vi "Update State Data.vi"(8 "error in (no error)":errorcluster, 9 "Data":variant, 10 "Argument":string, 11 "String Assertion in":refnum<class "String Assertion.lvclass">) -> (0 "error out":errorcluster, 3 "String Assertion out":refnum<class "String Assertion.lvclass">)   [LabVIEW 2020, in "MacroAssert.lvlib" / "String Assertion.lvclass"]
uses:
  String Assertion.lvclass
  String Assertion Type.ctl
  String Comparator.ctl
  Assertion Step/Assertion Step.lvclass
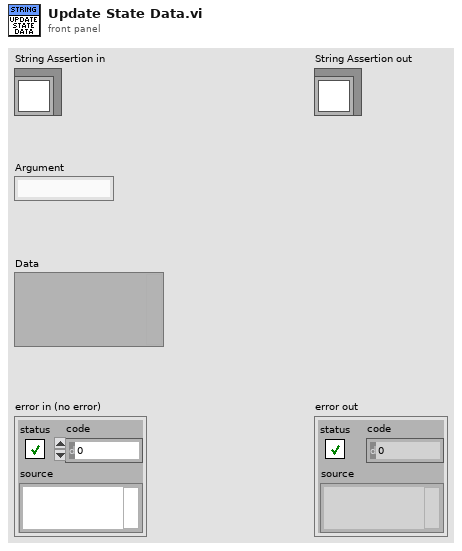
[diagram p1: front panel]
types:
  T1 = typedef "MacroAssert.lvlib/String Assertion.lvclass/String Assertion Type.ctl" = enum16{"String Ctl Value", "Ctl Caption Property", "Ctl Tip Strip Property", "Frontmost Window Name", "Frontmost VI Name"}
  T2 = typedef "MacroAssert.lvlib/String Assertion.lvclass/String Comparator.ctl" = enum16{"Contains", "Equals", "Starts with", "Ends with", "Does not contain", "Does not equal"}
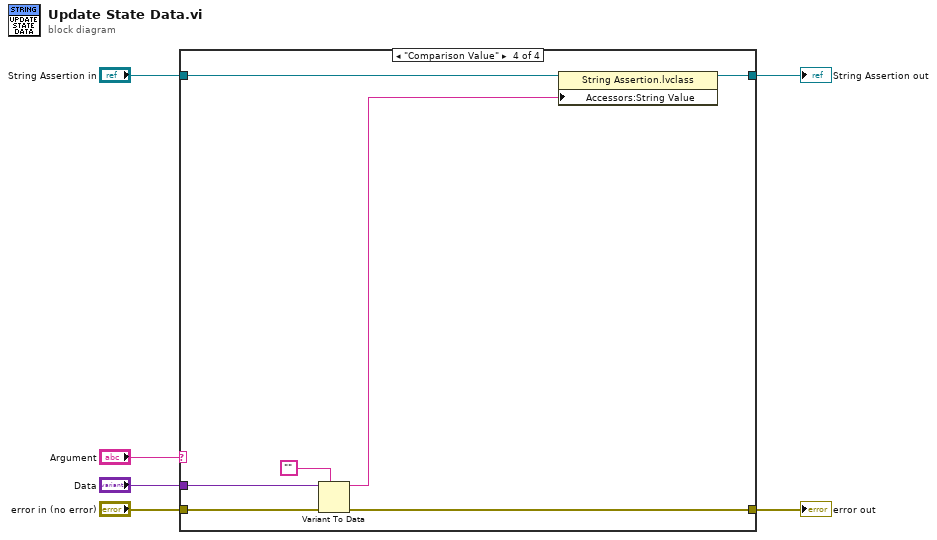
[diagram p0: block diagram]
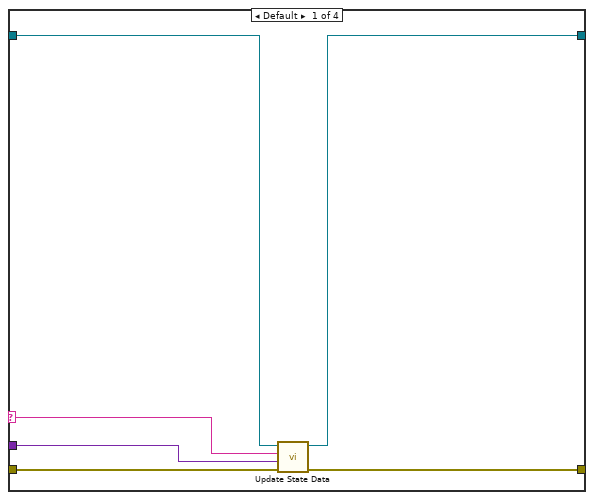
[diagram p2: hidden frame]
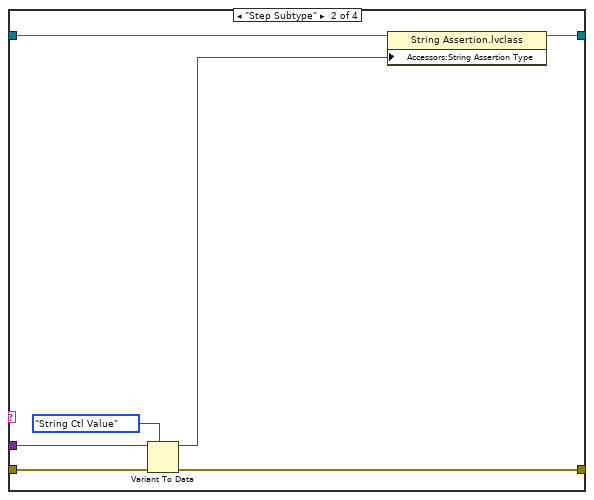
[diagram p3: hidden frame]
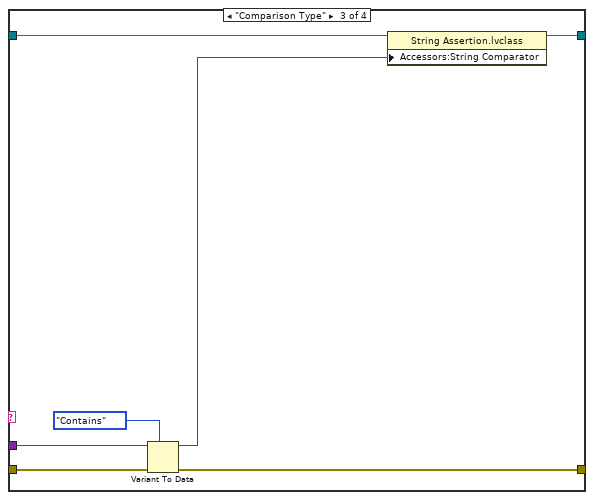
[diagram p4: hidden frame]
diagram:
  n1 = case shown="\"Comparison Value\"" "Argument" {
    selector: "Argument" -> [w9 _ _ _]
    tunnel: "String Assertion in" -> [w8 w19 w26 w33]
    tunnel: "error in (no error)" -> [w12 w17 w24 w31]
    tunnel: [w7 w18 w25 w32] -> w1
    tunnel: [w11 w16 w23 w30] -> w5
    tunnel: "Data" -> [w10 w14 w22 w29]
    frame Default {
      n2 = call-parent "Update State Data.vi"("error in (no error)"=w12, "Data"=w10, "Argument"=w9, "Assertion Step in"=w8) -> ("error out"=w11:errorcluster, "Assertion Step out"=w7:refnum<class "String Assertion.lvclass">)  [unwired: 6 in]
    }
    frame "Step Subtype" {
      n3 = Variant To Data(error in=w17, type=String_Assertion_Type."String Ctl Value" ("String Assertion Type"), Variant=w14) -> (data=w13:T1, error out=w16:errorcluster)
      n4 = property class="String Assertion.lvclass"(reference=w19, "Accessors:String Assertion Type"=w13) -> (reference out=w18:refnum<class "String Assertion.lvclass">)  [unwired: 1 in, 1 out]
    }
    frame "Comparison Type" {
      n5 = Variant To Data(error in=w24, type=String_Comparator."Contains" ("String Comparator"), Variant=w22) -> (data=w21:T2, error out=w23:errorcluster)
      n6 = property class="String Assertion.lvclass"(reference=w26, "Accessors:String Comparator"=w21) -> (reference out=w25:refnum<class "String Assertion.lvclass">)  [unwired: 1 in, 1 out]
    }
    frame "Comparison Value" {
      n7 = Variant To Data(error in=w31, type="", Variant=w29) -> (data=w28:string, error out=w30:errorcluster)
      n8 = property class="String Assertion.lvclass"(reference=w33, "Accessors:String Value"=w28) -> (reference out=w32:refnum<class "String Assertion.lvclass">)  [unwired: 1 in, 1 out]
    }
  }
  "error out" <- w5
  "String Assertion out" <- w1
